vi "XML Parse Parameters File.vi"(8 "error in":errorcluster, 11 "path to XML document":path caption="path to parameters xml") -> (0 "error out":errorcluster, 2 "Ports":T1[](array[typedef]) {"Labels"."Label (octal)" format="%o"})   [LabVIEW 2020, in "Ballard ARINC 429 System Explorer.lvlib" / "Implementation.lvlib"]
uses:
  Implementation.lvlib
  Types/XML Port.ctl
  Types/XML Label.ctl
  Types/XML Parameter.ctl
  Encoding and Decoding/Encoding.ctl
  96318c9f-5511-490f-8cf3-d6ae8ee7fbba.vi
  66ca86fd-bcc2-4251-bc28-8104269f3039.vi
  943041b1-b2f7-4370-bedb-ab00537ed944.vi
  6ae92e42-6cf0-49e1-9b75-7909647a45ce.vi
  adb928f7-1009-4efb-a5d9-0bfc5dee487e.vi
  7b08c8a5-aa6d-444a-b86a-d1c96e67564d.vi
  6672d625-2d78-4bdd-977b-59966d3b659c.vi
  22df0f7b-d61e-4401-8e57-e71f5e888b48.vi
  99e32819-dcb9-49ee-834c-aa385a1486ed.vi
  981bdbeb-0d03-4f18-aed9-4c0583961c72.vi
  e36fd712-4135-4e78-a029-16964563b434.vi
  425940f6-5d0f-474c-aa3a-0c20134fcdff.vi
  02f92bc1-6c4d-49ae-b9de-b575791265b9.vi
  42238a94-b246-4e7b-b757-40bd9f2bb64d.vi
  50c37b56-0bda-43fe-8735-dbe4ae60c9b2.vi
  96318c9f-5511-490f-8cf3-d6ae8ee7fbba.vi/2d82a847-c95d-455c-bd03-5e6a60b57ac1.vi
  99e32819-dcb9-49ee-834c-aa385a1486ed.vi/ccd9931e-42fe-4a7b-aad1-961e3c199a70.vi
  981bdbeb-0d03-4f18-aed9-4c0583961c72.vi/2d82a847-c95d-455c-bd03-5e6a60b57ac1.vi
  e36fd712-4135-4e78-a029-16964563b434.vi/2d82a847-c95d-455c-bd03-5e6a60b57ac1.vi
  02f92bc1-6c4d-49ae-b9de-b575791265b9.vi/ccd9931e-42fe-4a7b-aad1-961e3c199a70.vi
  42238a94-b246-4e7b-b757-40bd9f2bb64d.vi/ccd9931e-42fe-4a7b-aad1-961e3c199a70.vi
  <vilib>/xml/Load XML File.vi
  <vilib>/xml/NI_XML.lvlib
  <resource>/objmgr/DOMUserDefRef.rc
  Encoding and Decoding/Encoding and Decoding.lvlib
panel:
  out "parse errors":string
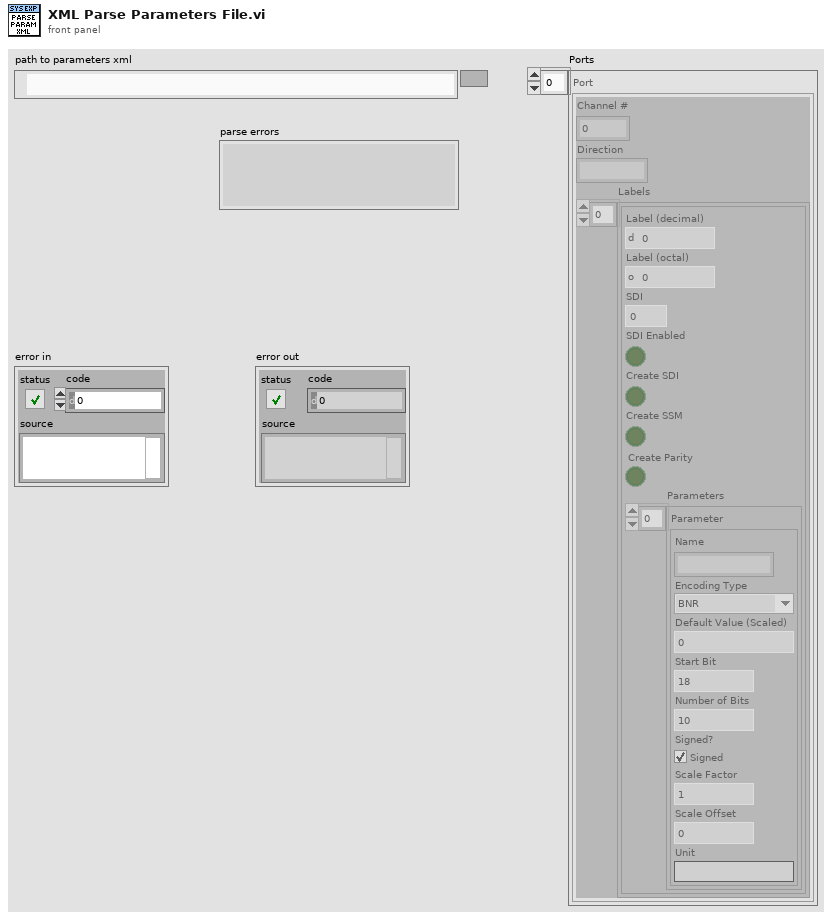
[diagram p1: front panel]
types:
  T1 = typedef "Ballard ARINC 429 System Explorer.lvlib/Implementation.lvlib/XML Port.ctl" = cluster{"Channel #":u16, "Direction":string, "Labels":T2[]}
  T2 = typedef "Ballard ARINC 429 System Explorer.lvlib/Implementation.lvlib/XML Label.ctl" = cluster{"Label (decimal)":i32, "Label (octal)":i32, "SDI":u8, "SDI Enabled":bool, "Create SDI":bool, "Create SSM":bool, "Create Parity":bool, "Parameters":T3[]}
  T3 = typedef "Ballard ARINC 429 System Explorer.lvlib/Implementation.lvlib/XML Parameter.ctl" = cluster{"Name":string, "Encoding Type":T4, "Default Value (Scaled)":dbl, "Start Bit":i32, "Number of Bits":i32, "Signed?":bool, "Scale Factor":dbl, "Scale Offset":dbl, "Unit":string}
  T4 = typedef "Encoding and Decoding.lvlib/Encoding.ctl" = enum16{"BNR", "BCD", "Discrete"}
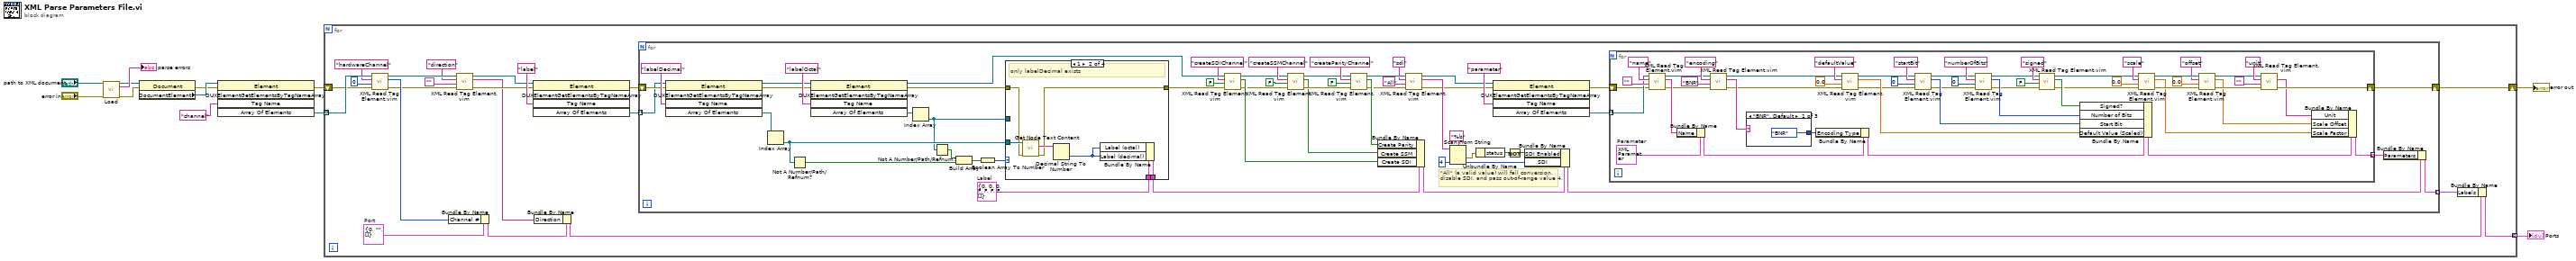
[diagram p0: block diagram]
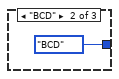
[diagram p2: hidden frame]
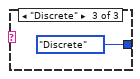
[diagram p3: hidden frame]
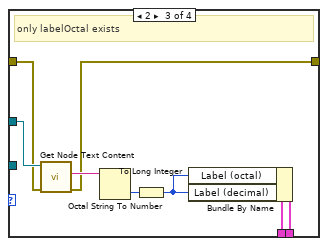
[diagram p5: hidden frame]
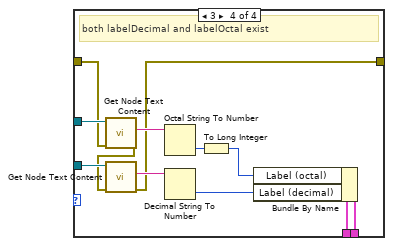
[diagram p6: hidden frame]
diagram:
  n1 = call-poly <vilib>:"Load.vi"("path to XML document"="path to XML document", "error in (no error)"="error in") -> ("DOM document out"=w7:refnum<k20>, "parse errors"=→"parse errors":string, "error out"=w1:errorcluster)  [unwired: 11 in]
  n2 = property class="Document"(reference=w7, error in=w1) -> (error out=w6:errorcluster, "DocumentElement"=w9:refnum<k20>)  [unwired: 1 out]
  n3 = invoke class="Element" method="DUXElementGetElementsByTagNameArray"(reference=w9, error in=w6, "Tag Name"="channel") -> (error out=w5:errorcluster, "Array Of Elements"=w8:refnum<k20>[])  [unwired: 2 in, 3 out]
  n4 = for {
    tunnel: w8 -> [w33] mode=indexing
    shift-right: [w28] -> w3
    shift-left: w5 -> [w19]
    tunnel: [w25] -> w4 mode=indexing
    w13 = T1 {"Channel #"=0, "Direction"="", "Labels"=[]}  # Port
    n5 = call "XML Read Tag Element.vim"("error in"=w19, "default"=u16 0, "Tag Name"="hardwareChannel", "node in"=w33) -> ("error out"=w17:errorcluster, "value"=w18:u16, "node out"=w23:refnum<k20>)  [unwired: 5 in]
    n6 = Bundle By Name(cluster=w13, "Channel #"=w18) -> (w32:T1)
    n7 = call "XML Read Tag Element.vim"("error in"=w17, "default"="", "Tag Name"="direction", "node in"=w23) -> ("error out"=w21:errorcluster, "value"=w20:string, "node out"=w24:refnum<k20>)  [unwired: 5 in]
    n8 = invoke class="Element" method="DUXElementGetElementsByTagNameArray"(reference=w24, error in=w21, "Tag Name"="label") -> (error out=w29:errorcluster, "Array Of Elements"=w30:refnum<k20>[])  [unwired: 2 in, 3 out]
    n9 = Bundle By Name(cluster=w32, "Direction"=w20) -> (w26:T1)
    n10 = for {
      tunnel: w30 -> [w83] mode=indexing
      shift-right: [w39] -> w28
      shift-left: w29 -> [w85]
      tunnel: [w35] -> w27 mode=indexing
      w34 = T2 {"Label (decimal)"=0, "Label (octal)"=0, "SDI"=0, "SDI Enabled"=FALSE, "Create SDI"=FALSE, "Create SSM"=FALSE, "Create Parity"=FALSE, "Parameters"=[]}  # Label
      # "\"All\" (a valid value) will fail conversion, disable SDI, and pass out-of-range value 4."
      n11 = invoke class="Element" method="DUXElementGetElementsByTagNameArray"(reference=w83, error in=w85, "Tag Name"="labelDecimal") -> (reference out=w80:refnum<k20>, error out=w79:errorcluster, "Array Of Elements"=w84:refnum<k20>[])  [unwired: 2 in, 2 out]
      n12 = Index Array(array=w84) -> (element=w74:refnum<k20>)  [unwired: 1 in]
      n13 = Not A Number/Path/Refnum?(number/path/refnum=w74) -> (NaN/Path/Refnum?=w77:bool)
      n14 = invoke class="Element" method="DUXElementGetElementsByTagNameArray"(reference=w80, error in=w79, "Tag Name"="labelOctal") -> (reference out=w70:refnum<k20>, error out=w72:errorcluster, "Array Of Elements"=w82:refnum<k20>[])  [unwired: 2 in, 2 out]
      n15 = Index Array(array=w82) -> (element=w73:refnum<k20>)  [unwired: 1 in]
      n16 = Not A Number/Path/Refnum?(number/path/refnum=w73) -> (NaN/Path/Refnum?=w78:bool)
      n17 = Build Array(w78, w77) -> (w76:bool[])
      n18 = Boolean Array To Number(Boolean array=w76) -> (number=w75:u32)
      n19 = case shown="1" w75 {
        tunnel: w34 -> [w143 w149 w157 w169]
        tunnel: [w143 w148 w156 w168] -> w69
        tunnel: w74 -> [_ w147 _ w165]
        tunnel: w73 -> [_ _ w154 w166]
        tunnel: w72 -> [w142 w145 w152 w161]
        tunnel: [w142 w144 w151 w159] -> w71
        frame 0, Default {
          # "neither labelDecimal or labelOctal exist"
        }
        frame 1 {
          # "only labelDecimal exists"
          n20 = call <vilib>:"Get Node Text Content.vi"("error in (no error)"=w145, "node in"=w147) -> ("error out"=w144:errorcluster, "node text"=w150:string)  [unwired: 7 in, 1 out]
          n21 = Decimal String To Number(string=w150) -> (number=w146:i32)  [unwired: 2 in, 1 out]
          n22 = Bundle By Name(cluster=w149, "Label (octal)"=w146, "Label (decimal)"=w146) -> (w148:T2)
        }
        frame 2 {
          # "only labelOctal exists"
          n23 = call <vilib>:"Get Node Text Content.vi"("error in (no error)"=w152, "node in"=w154) -> ("error out"=w151:errorcluster, "node text"=w158:string)  [unwired: 7 in, 1 out]
          n24 = Octal String To Number(4:w158) -> (0:w155:u32)  [unwired: 2 in, 1 out]
          n25 = To Long Integer(number=w155) -> (32bit integer=w153:i32)
          n26 = Bundle By Name(cluster=w157, "Label (octal)"=w153, "Label (decimal)"=w153) -> (w156:T2)
        }
        frame 3 {
          # "both labelDecimal and labelOctal exist"
          n27 = call <vilib>:"Get Node Text Content.vi"("error in (no error)"=w161, "node in"=w166) -> ("error out"=w160:errorcluster, "node text"=w167:string)  [unwired: 7 in, 1 out]
          n28 = call <vilib>:"Get Node Text Content.vi"("error in (no error)"=w160, "node in"=w165) -> ("error out"=w159:errorcluster, "node text"=w170:string)  [unwired: 7 in, 1 out]
          n29 = Octal String To Number(4:w167) -> (0:w163:u32)  [unwired: 2 in, 1 out]
          n30 = Decimal String To Number(string=w170) -> (number=w164:i32)  [unwired: 2 in, 1 out]
          n31 = To Long Integer(number=w163) -> (32bit integer=w162:i32)
          n32 = Bundle By Name(cluster=w169, "Label (octal)"=w162, "Label (decimal)"=w164) -> (w168:T2)
        }
      }
      n33 = call "XML Read Tag Element.vim"("error in"=w71, "default"=FALSE, "Tag Name"="createSDIChannel", "node in"=w70) -> ("error out"=w63:errorcluster, "value"=w67:bool, "node out"=w64:refnum<k20>)  [unwired: 5 in]
      n34 = call "XML Read Tag Element.vim"("error in"=w63, "default"=FALSE, "Tag Name"="createSSMChannel", "node in"=w64) -> ("error out"=w62:errorcluster, "value"=w60:bool, "node out"=w61:refnum<k20>)  [unwired: 5 in]
      n35 = call "XML Read Tag Element.vim"("error in"=w62, "default"=FALSE, "Tag Name"="createParityChannel", "node in"=w61) -> ("error out"=w52:errorcluster, "value"=w59:bool, "node out"=w55:refnum<k20>)  [unwired: 5 in]
      n36 = Bundle By Name(cluster=w69, "Create Parity"=w59, "Create SSM"=w60, "Create SDI"=w67) -> (w54:T2)
      n37 = call "XML Read Tag Element.vim"("error in"=w52, "default"="All", "Tag Name"="sdi", "node in"=w55) -> ("error out"=w42:errorcluster, "value"=w44:string, "node out"=w41:refnum<k20>)  [unwired: 5 in]
      n38 = Scan From String(format string="%b", input string=w44, default 1=u8 4 ("default value 1")) -> (error out=w47:errorcluster, output 1=w48:u8)  [unwired: 2 in, 2 out]
      n39 = Unbundle By Name(w47) -> ("status"=w46:bool)
      n40 = invoke class="Element" method="DUXElementGetElementsByTagNameArray"(reference=w41, error in=w42, "Tag Name"="parameter") -> (error out=w40:errorcluster, "Array Of Elements"=w38:refnum<k20>[])  [unwired: 2 in, 3 out]
      n41 = Not(x=w46) -> (.not. x?=w45:bool)
      n42 = Bundle By Name(cluster=w54, "SDI Enabled"=w45, "SDI"=w48) -> (w36:T2)
      n43 = for {
        shift-right: [w92] -> w39
        shift-left: w40 -> [w135]
        tunnel: w38 -> [w136] mode=indexing
        tunnel: [w90] -> w37 mode=indexing
        w120 = T3 {"Name"="", "Encoding Type"=enum."BNR", "Default Value (Scaled)"=0.0, "Start Bit"=8, "Number of Bits"=1, "Signed?"=FALSE, "Scale Factor"=1.0, "Scale Offset"=0.0, "Unit"=""}  # Parameter
        n44 = call "XML Read Tag Element.vim"("error in"=w135, "default"="", "Tag Name"="name", "node in"=w136) -> ("error out"=w130:errorcluster, "value"=w134:string, "node out"=w131:refnum<k20>)  [unwired: 5 in]
        n45 = Bundle By Name(cluster=w120, "Name"=w134) -> (w129:T3)
        n46 = call "XML Read Tag Element.vim"("error in"=w130, "default"="BNR", "Tag Name"="encoding", "node in"=w131) -> ("error out"=w123:errorcluster, "value"=w127:string, "node out"=w124:refnum<k20>)  [unwired: 5 in]
        n47 = case shown="\"BNR\", Default" w127 {
          tunnel: [Encoding."BNR" ("Encoding Type") Encoding."BCD" ("Encoding Type") Encoding."Discrete" ("Encoding Type")] -> w128
          frame "BNR", Default {
          }
          frame "BCD" {
          }
          frame "Discrete" {
          }
        }
        n48 = Bundle By Name(cluster=w129, "Encoding Type"=w128) -> (w121:T3)
        n49 = call "XML Read Tag Element.vim"("error in"=w123, "default"=0.0, "Tag Name"="defaultValue", "node in"=w124) -> ("error out"=w111:errorcluster, "value"=w122:dbl, "node out"=w117:refnum<k20>)  [unwired: 5 in]
        n50 = call "XML Read Tag Element.vim"("error in"=w111, "default"=0, "Tag Name"="startBit", "node in"=w117) -> ("error out"=w110:errorcluster, "value"=w113:i32, "node out"=w114:refnum<k20>)  [unwired: 5 in]
        n51 = call "XML Read Tag Element.vim"("error in"=w110, "default"=0, "Tag Name"="numberOfBits", "node in"=w114) -> ("error out"=w106:errorcluster, "value"=w112:i32, "node out"=w107:refnum<k20>)  [unwired: 5 in]
        n52 = call "XML Read Tag Element.vim"("error in"=w106, "default"=FALSE, "Tag Name"="signed", "node in"=w107) -> ("error out"=w97:errorcluster, "value"=w105:bool, "node out"=w98:refnum<k20>)  [unwired: 5 in]
        n53 = Bundle By Name(cluster=w121, "Signed?"=w105, "Number of Bits"=w112, "Start Bit"=w113, "Default Value (Scaled)"=w122) -> (w91:T3)
        n54 = call "XML Read Tag Element.vim"("error in"=w97, "default"=0.0, "Tag Name"="scale", "node in"=w98) -> ("error out"=w104:errorcluster, "value"=w89:dbl, "node out"=w103:refnum<k20>)  [unwired: 5 in]
        n55 = call "XML Read Tag Element.vim"("error in"=w104, "default"=0.0, "Tag Name"="offset", "node in"=w103) -> ("error out"=w93:errorcluster, "value"=w88:dbl, "node out"=w94:refnum<k20>)  [unwired: 5 in]
        n56 = call "XML Read Tag Element.vim"("error in"=w93, "default"="", "Tag Name"="unit", "node in"=w94) -> ("error out"=w92:errorcluster, "value"=w87:string)  [unwired: 5 in, 1 out]
        n57 = Bundle By Name(cluster=w91, "Unit"=w87, "Scale Offset"=w88, "Scale Factor"=w89) -> (w90:T3)
      }
      n58 = Bundle By Name(cluster=w36, "Parameters"=w37) -> (w35:T2)
    }
    n59 = Bundle By Name(cluster=w26, "Labels"=w27) -> (w25:T1)
  }
  "Ports" <- w4
  "error out" <- w3
